vi "Pixel Size.vi"(8 "error in (no error)":errorcluster caption="entrée d'erreur (pas d'erreur)", 11 "Acq Cam Basler en entrée":refnum<class "Acq Cam Basler.lvclass">) -> (0 "error out":errorcluster caption="sortie d'erreur", 3 "Acq Cam Basler en sortie":refnum<class "Acq Cam Basler.lvclass">)   [LabVIEW 2023, in "Acq Cam Basler.lvclass"]
uses:
  Acq Cam Basler.lvclass
  C:/Program Files (x86)/National Instruments/LabVIEW 2023/vi.lib/addons/_Workers/Library/Classes/Worker/Worker.lvclass
  Acq Cam Basler.lvclass/Acq Cam Basler.ctl
  <vilib>/addons/_Workers/Library/Classes/Message/Enqueue Message to Queue.vi
  <vilib>/addons/_Workers/Library/Classes/Message/Message.lvclass
  UI Cam Basler/UI Cam Basler.lvclass
  C:/Program Files (x86)/National Instruments/LabVIEW 2023/vi.lib/addons/_Workers/Library/Classes/Workers Object/Workers Object.lvclass
  C:/Users/flepetit/Desktop/CamView-mdi-LV/Workers/Acq Cam Basler/Acq Cam Basler.lvclass
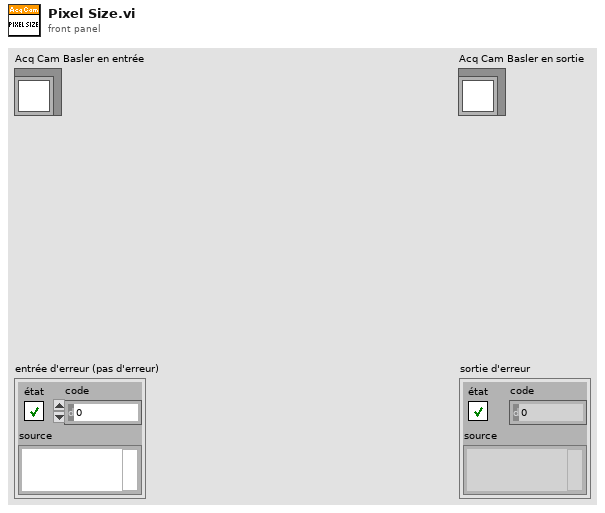
[diagram p1: front panel]
types:
  T1 = typedef "Workers.lvlib/Case Label.ctl" = string
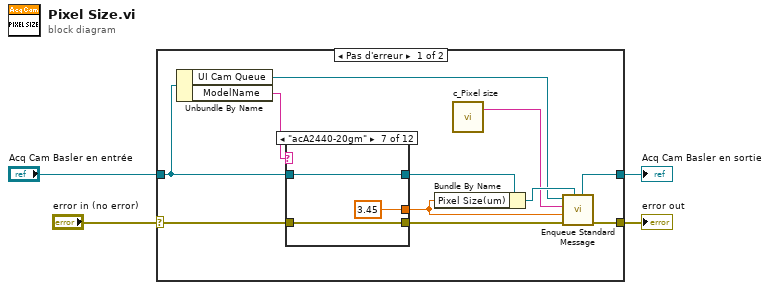
[diagram p0: block diagram]
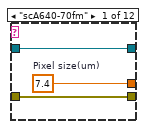
[diagram p2: hidden frame]
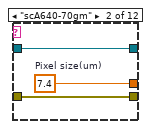
[diagram p3: hidden frame]
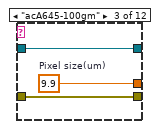
[diagram p4: hidden frame]
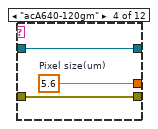
[diagram p5: hidden frame]
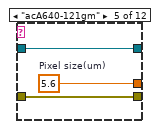
[diagram p6: hidden frame]
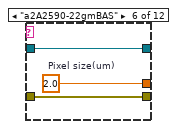
[diagram p7: hidden frame]
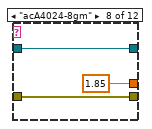
[diagram p8: hidden frame]
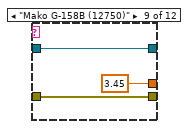
[diagram p9: hidden frame]
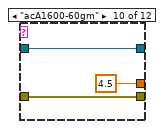
[diagram p10: hidden frame]
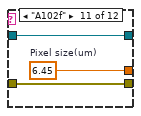
[diagram p11: hidden frame]
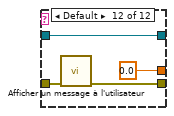
[diagram p12: hidden frame]
diagram:
  n1 = case shown="Pas d'erreur" "error in (no error)" {
    selector: "error in (no error)" -> [w14 w54]
    tunnel: [w8 w54] -> w3
    tunnel: [w10 w53] -> w1
    tunnel: "Acq Cam Basler en entrée" -> [w12 w53]
    frame No Error {
      n2 = Unbundle By Name(w12) -> ("UI Cam Queue"=w6:refnum<class "Message Queue.lvclass">, "ModelName"=w15:string)
      n3 = case shown="\"acA2440-20gm\"" w15 {
        tunnel: [w18 w21 w24 w27 w30 w33 3.45 ("Pixel size(um)") 1.85 ("Pixel size(um)") 3.45 ("Pixel size(um)") 4.5 ("Pixel size(um)") w48 0.0 ("Pixel size(um)")] -> w5
        tunnel: [w17 w20 w23 w26 w29 w32 w35 w38 w41 w44 w47 w49] -> w9
        tunnel: w14 -> [w17 w20 w23 w26 w29 w32 w35 w38 w41 w44 w47 w50]
        tunnel: [w16 w19 w22 w25 w28 w31 w34 w37 w40 w43 w46 w51] -> w13
        tunnel: w12 -> [w16 w19 w22 w25 w28 w31 w34 w37 w40 w43 w46 w51]
        frame "scA640-70fm" {
          w18 = 7.4  # Pixel size(um)
        }
        frame "scA640-70gm" {
          w21 = 7.4  # Pixel size(um)
        }
        frame "acA645-100gm" {
          w24 = 9.9  # Pixel size(um)
        }
        frame "acA640-120gm" {
          w27 = 5.6  # Pixel size(um)
        }
        frame "acA640-121gm" {
          w30 = 5.6  # Pixel size(um)
        }
        frame "a2A2590-22gmBAS" {
          w33 = 2.0  # Pixel size(um)
        }
        frame "acA2440-20gm" {
        }
        frame "acA4024-8gm" {
        }
        frame "Mako G-158B (12750)" {
        }
        frame "acA1600-60gm" {
        }
        frame "A102f" {
          w48 = 6.45  # Pixel size(um)
        }
        frame Default {
          n4 = call "Afficher un message à l'utilisateur"("error in (no error)"=w50) -> ("error out"=w49:errorcluster)  [unwired: 9 in, 1 out]
        }
      }
      n5 = Bundle By Name(cluster=w13, "Pixel Size(um)"=w5) -> (w11:refnum<class "Acq Cam Basler.lvclass">)
      n6 = call "c_Pixel size.vi"() -> ("Case Label"=w7:T1)  [unwired: 1 in]
      n7 = call-poly <vilib>:"Enqueue Standard Message.vi"("Worker"=w11, "error in"=w9, "Data"=w5, "Case Label"=w7, "Message Queue"=w6) -> ("error out"=w8:errorcluster, "dup Worker out"=w10:refnum<class "Acq Cam Basler.lvclass">)  [unwired: 4 in, 1 out]
    }
    frame Error {
    }
  }
  "error out" <- w3
  "Acq Cam Basler en sortie" <- w1
